vi "Decompose Cluster - String - Element Value.vi"() -> ()   [LabVIEW 2017, in "Composition.Tests.lvlib"]
uses:
  Composition.Tests.lvlib
  Composition/Composition.lvlib
  <vilib>/addons/_JKI Toolkits/Caraya/classes/Assert/Assert.lvclass
  <vilib>/addons/_JKI Toolkits/Caraya/classes/Test/Test.lvclass
panel:
  out "error out":errorcluster
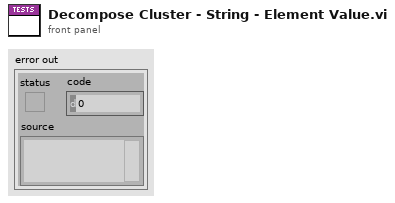
[diagram p1: front panel]
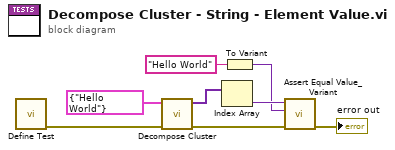
[diagram p0: block diagram]
diagram:
  n1 = call <vilib>:"Define Test.vi"() -> ("error out"=w1:errorcluster)  [unwired: 11 in]
  n2 = call "Decompose Cluster.vi"("error in (no error)"=w1, "Cluster"=cluster{string} {"Hello World"}) -> ("error out"=w7:errorcluster, "Cluster Elements"=w6:variant[])  [unwired: 8 in]
  n3 = Index Array(array=w6) -> (element=w3:variant)  [unwired: 1 in]
  n4 = To Variant(anything="Hello World") -> (Variant=w2:variant)
  n5 = call <vilib>:"Assert Equal Value_Variant.vi"("error in (no error)"=w7, "Y"=w2, "X"=w3) -> ("error out"=→"error out":errorcluster)  [unwired: 8 in]
